vi "Track Info FGV.vi"(7 "Track Info FGV Enum":T1, 8 "error in (no error)":errorcluster, 9 "Multiple Track Info In":T2[](array[typedef]), 10 "Track Info In":T2, 11 "Track Path":path) -> (0 "error out":errorcluster, 1 "Multiple Track Info Out":T2[](array[typedef]), 2 "Track Info Out":T2, 3 "Track Info Found?":bool)   [LabVIEW 2018, in "Track Info.lvlib"]
uses:
  Track Info.lvlib
  Track Info.ctl
  Track Info FGV Enum.ctl
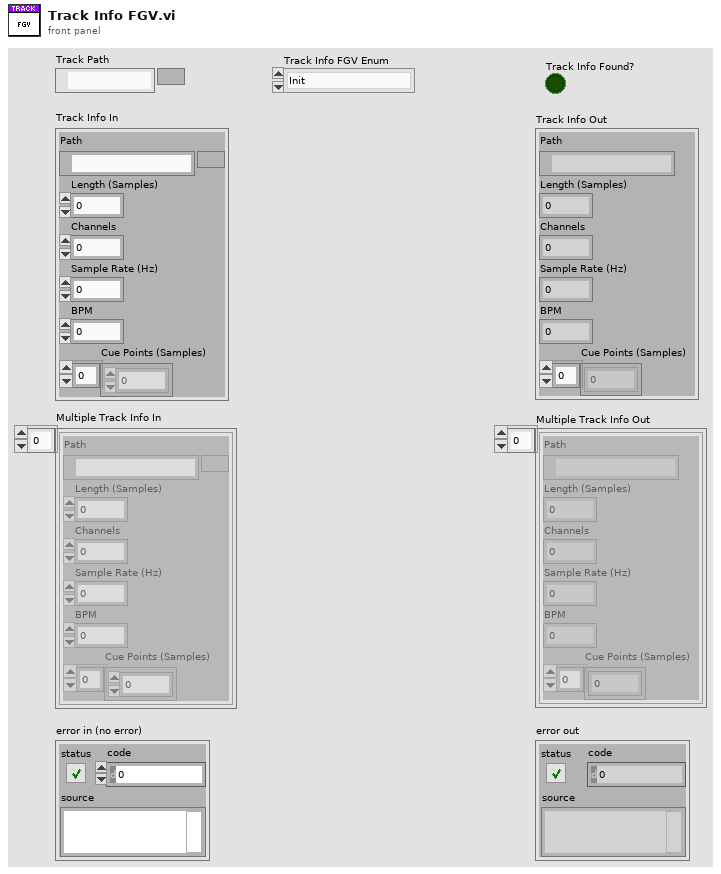
[diagram p1: front panel]
types:
  T1 = typedef "Track Info.lvlib/Track Info FGV Enum.ctl" = enum16{"Init", "Update Track", "Update Multiple Tracks", "Get Track", "Get Multiple Tracks"}
  T2 = typedef "Track Info.lvlib/Track Info.ctl" = cluster{"Path":path, "Length (Samples)":i32, "Channels":i32, "Sample Rate (Hz)":i32, "BPM":dbl, "Cue Points (Samples)":i32[]}
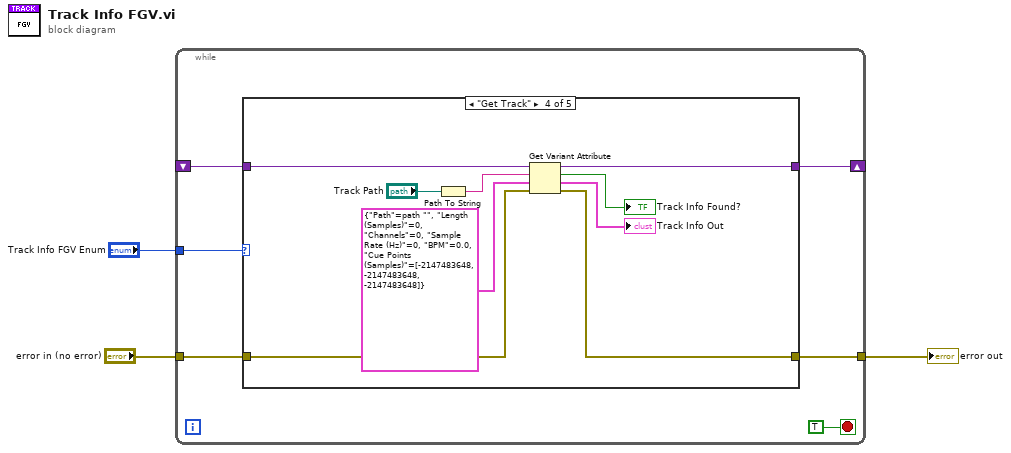
[diagram p0: block diagram]
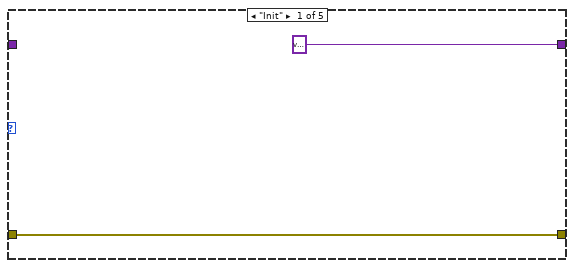
[diagram p2: hidden frame]
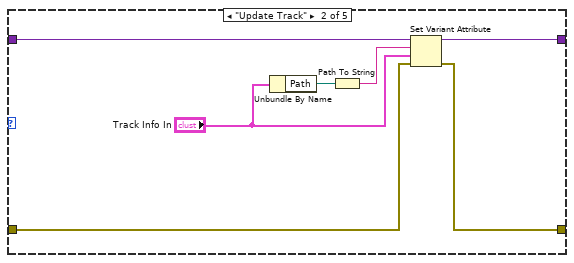
[diagram p3: hidden frame]
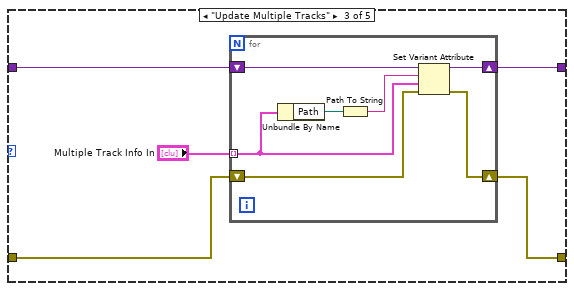
[diagram p4: hidden frame]
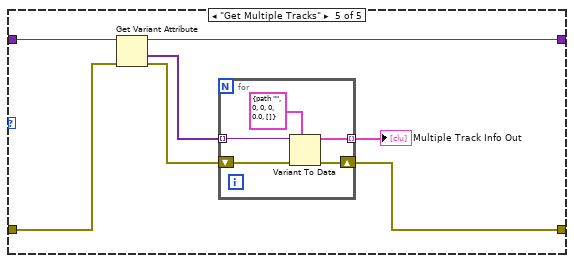
[diagram p5: hidden frame]
diagram:
  n1 = while {
    shift-right: [w9] -> _
    shift-left: _ -> [w8]
    tunnel: "Track Info FGV Enum" -> [w7]
    tunnel: "error in (no error)" -> [w5]
    tunnel: [w4] -> w1
    stop <- TRUE stop-if-true
    n2 = case shown="\"Get Track\"" w7 {
      tunnel: [variant w14 w22 w35 w44] -> w9
      tunnel: w8 -> [_ w18 w23 w39 w46]
      tunnel: w5 -> [w10 w13 w20 w32 w42]
      tunnel: [w10 w12 w19 w31 w40] -> w4
      frame "Init" {
      }
      frame "Update Track" {
        n3 = Unbundle By Name("Track Info In") -> ("Path"=w17:path)
        n4 = Path To String(path=w17) -> (string=w16:string)
        n5 = Set Variant Attribute(Variant=w18, name=w16, value="Track Info In", error in=w13) -> (Variant out=w14:variant, error out=w12:errorcluster)  [unwired: 1 out]
      }
      frame "Update Multiple Tracks" {
        n6 = for {
          tunnel: "Multiple Track Info In" -> [w26] mode=indexing
          shift-right: [w27] -> w22
          shift-left: w23 -> [w30]
          shift-right: [w24] -> w19
          shift-left: w20 -> [w25]
          n7 = Unbundle By Name(w26) -> ("Path"=w29:path)
          n8 = Path To String(path=w29) -> (string=w28:string)
          n9 = Set Variant Attribute(Variant=w30, name=w28, value=w26, error in=w25) -> (Variant out=w27:variant, error out=w24:errorcluster)  [unwired: 1 out]
        }
      }
      frame "Get Track" {
        n10 = Path To String(path="Track Path") -> (string=w36:string)
        n11 = Get Variant Attribute(Variant=w39, name=w36, default value (empty Variant)=T2 {"Path"=path "", "Length (Samples)"=0, "Channels"=0, "Sample Rate (Hz)"=0, "BPM"=0.0, "Cue Points (Samples)"=[-2147483648, -2147483648, -2147483648]} ("Track Info"), error in=w32) -> (duplicate Variant=w35:variant, found=→"Track Info Found?":bool, value=→"Track Info Out":T2, error out=w31:errorcluster)
      }
      frame "Get Multiple Tracks" {
        n12 = Get Variant Attribute(Variant=w46, error in=w42) -> (duplicate Variant=w44:variant, values=w45:variant[], error out=w41:errorcluster)  [unwired: 2 in, 1 out]
        n13 = for {
          tunnel: w45 -> [w51] mode=indexing
          tunnel: [w49] -> w43 mode=indexing
          shift-right: [w47] -> w40
          shift-left: w41 -> [w48]
          n14 = Variant To Data(error in=w48, type=T2 {"Path"=path "", "Length (Samples)"=0, "Channels"=0, "Sample Rate (Hz)"=0, "BPM"=0.0, "Cue Points (Samples)"=[]} ("Track Info"), Variant=w51) -> (data=w49:T2, error out=w47:errorcluster)
        }
        "Multiple Track Info Out" <- w43
      }
    }
  }
  "error out" <- w1
